vi "To Byte Array (EEPROM Header).vi"(1 "EEPROM Header":T1={"Checksum"=0, "Product Code"=0, "Hardware Current Version"=0, "Hardware Oldest Compatible Version"=0, "EEPROM Map Current Version"=0, "EEPROM Map Oldest Compatible Version"=0, "User Password"="", "Pointer to Factory Header"=0, "Pointer to User Header"=0, "Recommended Interval"=0, "Number of Reserved Bytes"=32} {"Product Code" format="%x"; "Checksum" format="%x"}) -> (0 "byte array out":u8[](array[numeric]) format="%x")   [LabVIEW 2015, in "ni579x Config v2 Shared.lvlib"]
uses:
  <instrlib>/ni579x/Config/v2/Shared/ni579x Config v2 Shared.lvlib
  <instrlib>/ni579x/Config/v2/Shared/Types/EEPROM/ni579x EEPROM Header.ctl
  <instrlib>/ni579x/Config/v2/Shared/Conversions/To Byte Array (U16).vi
  <instrlib>/ni579x/Config/v2/Shared/Conversions/To Byte Array (U32).vi
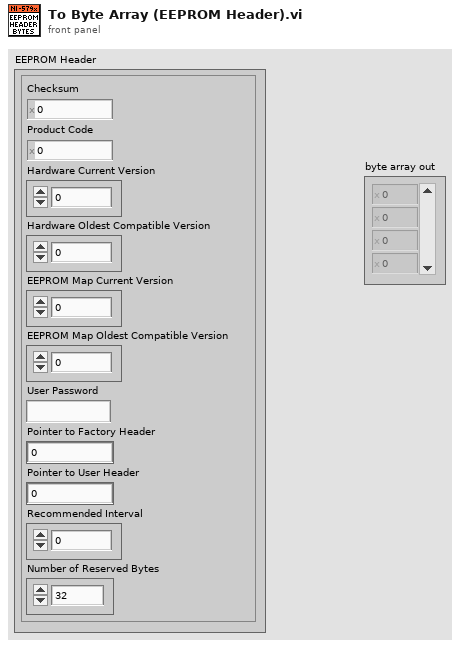
[diagram p1: front panel]
types:
  T1 = typedef "ni579x Config v2 Shared.lvlib/ni579x EEPROM Header.ctl" = cluster{"Checksum":u32, "Product Code":u16, "Hardware Current Version":u16, "Hardware Oldest Compatible Version":u16, "EEPROM Map Current Version":u16, "EEPROM Map Oldest Compatible Version":u16, "User Password":string, "Pointer to Factory Header":u32, "Pointer to User Header":u32, "Recommended Interval":u16, "Number of Reserved Bytes":i32}
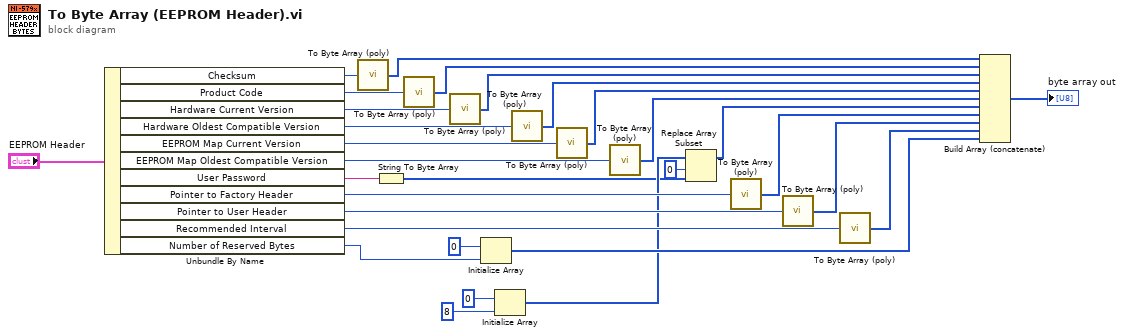
[diagram p0: block diagram]
diagram:
  n1 = Unbundle By Name("EEPROM Header") -> ("Checksum"=w30:u32, "Product Code"=w29:u16, "Hardware Current Version"=w28:u16, "Hardware Oldest Compatible Version"=w27:u16, "EEPROM Map Current Version"=w26:u16, "EEPROM Map Oldest Compatible Version"=w25:u16, "User Password"=w5:string, "Pointer to Factory Header"=w24:u32, "Pointer to User Header"=w23:u32, "Recommended Interval"=w22:u16, "Number of Reserved Bytes"=w20:i32)
  n2 = call-poly <instrlib>:"To Byte Array (poly).vi"("element in"=w30) -> ("byte array out"=w19:u8[])
  n3 = String To Byte Array(string=w5) -> (unsigned byte array=w2:u8[])
  n4 = call-poly <instrlib>:"To Byte Array (poly).vi"("element in"=w29) -> ("byte array out"=w18:u8[])
  n5 = call-poly <instrlib>:"To Byte Array (poly).vi"("element in"=w28) -> ("byte array out"=w17:u8[])
  n6 = Initialize Array(u8 0, w20) -> (w10:u8[])
  n7 = Initialize Array(u8 0, 8 ("dimension size")) -> (w4:u8[])
  n8 = call-poly <instrlib>:"To Byte Array (poly).vi"("element in"=w27) -> ("byte array out"=w16:u8[])
  n9 = call-poly <instrlib>:"To Byte Array (poly).vi"("element in"=w26) -> ("byte array out"=w15:u8[])
  n10 = call-poly <instrlib>:"To Byte Array (poly).vi"("element in"=w25) -> ("byte array out"=w14:u8[])
  n11 = Replace Array Subset(array=w4, new element=w2, index=0) -> (w1:u8[])
  n12 = call-poly <instrlib>:"To Byte Array (poly).vi"("element in"=w24) -> ("byte array out"=w13:u8[])
  n13 = call-poly <instrlib>:"To Byte Array (poly).vi"("element in"=w23) -> ("byte array out"=w12:u8[])
  n14 = call-poly <instrlib>:"To Byte Array (poly).vi"("element in"=w22) -> ("byte array out"=w11:u8[])
  n15 = Build Array (concatenate)(w19, w18, w17, w16, w15, w14, w1, w13, w12, w11, w10) -> (→"byte array out":u8[])
